vi "BusB Align Packet.vi"(8 "error in":errorcluster, 10 "String In":string, 11 "VISA resource in":refnum<visa-resource-name>) -> (0 "error out":errorcluster, 1 "Match & Update":bool, 2 "String Out":string, 3 "VISA resource out":refnum<visa-resource-name>)   [LabVIEW 2016, in "Impedance Data Acquisition and Decoding.lvlib"]
uses:
  Impedance Data Acquisition and Decoding.lvlib
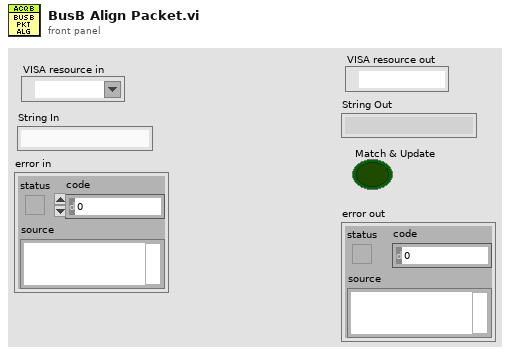
[diagram p1: front panel]
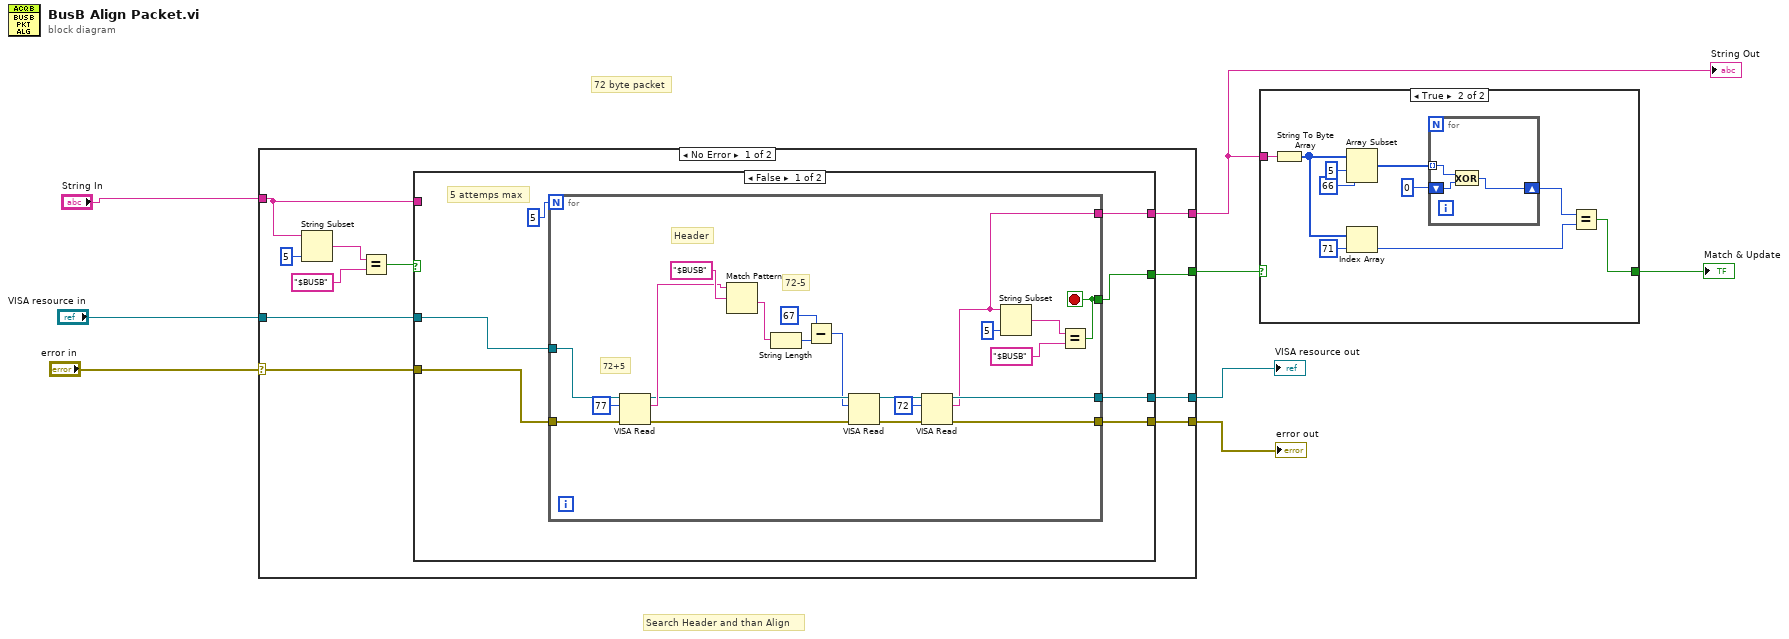
[diagram p0: block diagram]
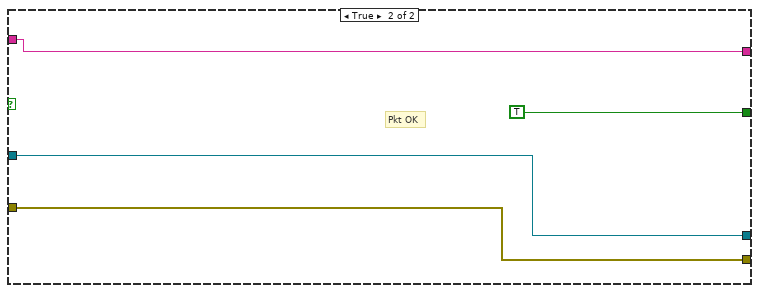
[diagram p3: hidden frame]
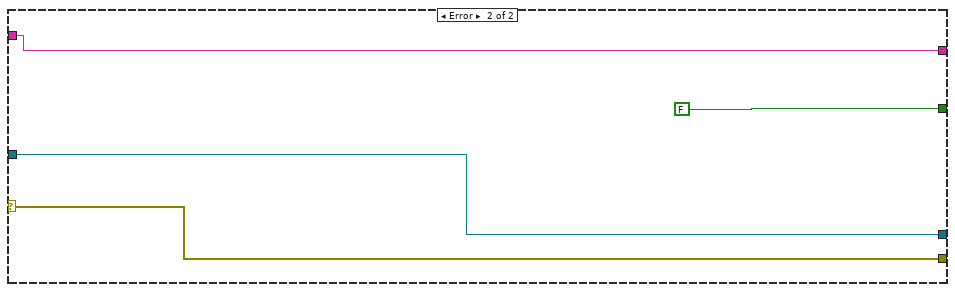
[diagram p4: hidden frame]
diagram:
  # "Search Header and than Align"
  # "72 byte packet"
  n1 = case shown="No Error" "error in" {
    selector: "error in" -> [w17 w55]
    tunnel: [w11 FALSE] -> w1
    tunnel: [w19 w54] -> w8
    tunnel: [w18 w55] -> w7
    tunnel: "VISA resource in" -> [w16 w54]
    tunnel: "String In" -> [w10 w52]
    tunnel: [w9 w52] -> w3
    frame No Error {
      n2 = String Subset(string=w10, length (rest)=5 ("length (rest)")) -> (substring=w14:string)  [unwired: 1 in]
      n3 = Equal?(x=w14, y="$BUSB" ("regular expression")) -> (x = y?=w12:bool)
      n4 = case shown="False" w12 {
        tunnel: [w26 w51] -> w19
        tunnel: [w25 w50] -> w18
        tunnel: w17 -> [w23 w50]
        tunnel: w16 -> [w22 w51]
        tunnel: [w21 TRUE] -> w11
        tunnel: w10 -> [_ w48]
        tunnel: [w20 w48] -> w9
        frame False {
          # "5 attemps max"
          n5 = for {
            N: 5 -> [_]
            tunnel: w23 -> [w47]
            tunnel: [w33] -> w26
            tunnel: [w32] -> w25
            tunnel: w22 -> [w45]
            tunnel: [w28] -> w21
            tunnel: [w27] -> w20
            stop <- w28 stop-if-true
            # "Header"
            # "72-5"
            # "72+5"
            n6 = VISA Read(VISA resource name=w45, byte count=u32 77, error in (no error)=w47) -> (VISA resource name out=w38:refnum<visa-resource-name>, read buffer=w42:string, error out=w46:errorcluster)  [unwired: 1 out]
            n7 = Match Pattern(string=w42, regular expression="$BUSB") -> (after substring=w41:string)  [unwired: 1 in, 3 out]
            n8 = String Length(string=w41) -> (length=w40:i32)
            n9 = Subtract(x=67, y=w40) -> (x-y=w37:i32)
            n10 = VISA Read(VISA resource name=w38, byte count=w37, error in (no error)=w46) -> (VISA resource name out=w36:refnum<visa-resource-name>, error out=w35:errorcluster)  [unwired: 2 out]
            n11 = VISA Read(VISA resource name=w36, byte count=u32 72, error in (no error)=w35) -> (VISA resource name out=w33:refnum<visa-resource-name>, read buffer=w27:string, error out=w32:errorcluster)  [unwired: 1 out]
            n12 = String Subset(string=w27, length (rest)=5 ("length (rest)")) -> (substring=w30:string)  [unwired: 1 in]
            n13 = Equal?(x=w30, y="$BUSB" ("regular expression")) -> (x = y?=w28:bool)
          }
        }
        frame True {
          # "Pkt OK"
        }
      }
    }
    frame Error {
    }
  }
  "VISA resource out" <- w8
  "error out" <- w7
  "String Out" <- w3
  n14 = case shown="True" w1 {
    selector: w1 -> [w56 _]
    tunnel: [w56 w57] -> w2
    tunnel: w3 -> [_ w66]
    frame False {
      # "Already Invalid Packet\nIgnore"
    }
    frame True {
      n15 = String To Byte Array(string=w66) -> (unsigned byte array=w63:u8[])
      n16 = Array Subset(array=w63, index=5, length=66) -> (w61:u8[])
      n17 = Index Array(array=w63, index=71) -> (element=w58:u8)
      n18 = for {
        tunnel: w61 -> [w68] mode=indexing
        shift-right: [w67] -> w59
        shift-left: u8 0 -> [w69]
        n19 = Exclusive Or(1:w69, 2:w68) -> (0:w67:u8)
      }
      n20 = Equal?(x=w59, y=w58) -> (x = y?=w57:bool)
    }
  }
  "Match & Update" <- w2
